vi "Read ODrive return data.vi"(8 "error in (no error)":errorcluster, 11 "Refnum in":refnum<k20>) -> (0 "error out":errorcluster, 3 "Refnum out":refnum<k20>)   [LabVIEW 2016]
uses:
  <vilib>/Utility/error.llb/Error Cluster From Error Code.vi
  <vilib>/RVI Host/nirviSupport.llb/nirviErrorClusterFromErrorCode.vi
  <vilib>/rvi/errors/niLvFpgaAdjustHostInterfaceError.vi
  Shared resoruces/ODrive State and Info.vi
  Shared resoruces/Navigation Variables.vi
  <vilib>/rvi/interface/nirviMethod/nirviMethod.xnode
  <vilib>/ErrorRing/Error Ring.xnode
  <vilib>/rvi/interface/nirviReadWriteControl/nirviReadWriteControl.xnode
  Shared resoruces/Shared resources RT.lvlib
  NiFpgaLv.dll
  <vilib>/rvi/interface/Simulation/niFpgaSimulationCallBeginRW.vi
  <vilib>/FPGAPlugInAG/Dynamic/niLvFpga_AcknowledgeIrq_Dynamic.vi
  <vilib>/rvi/interface/nirviMethod/StockFPGA_InlinedMethodWaitForSingleIRQ.vi
  <vilib>/FPGAPlugInAG/Dynamic/niLvFpga_WaitOnIrq_Dynamic.vi
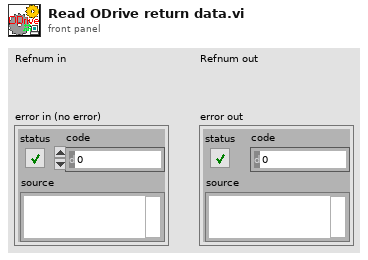
[diagram p1: front panel]
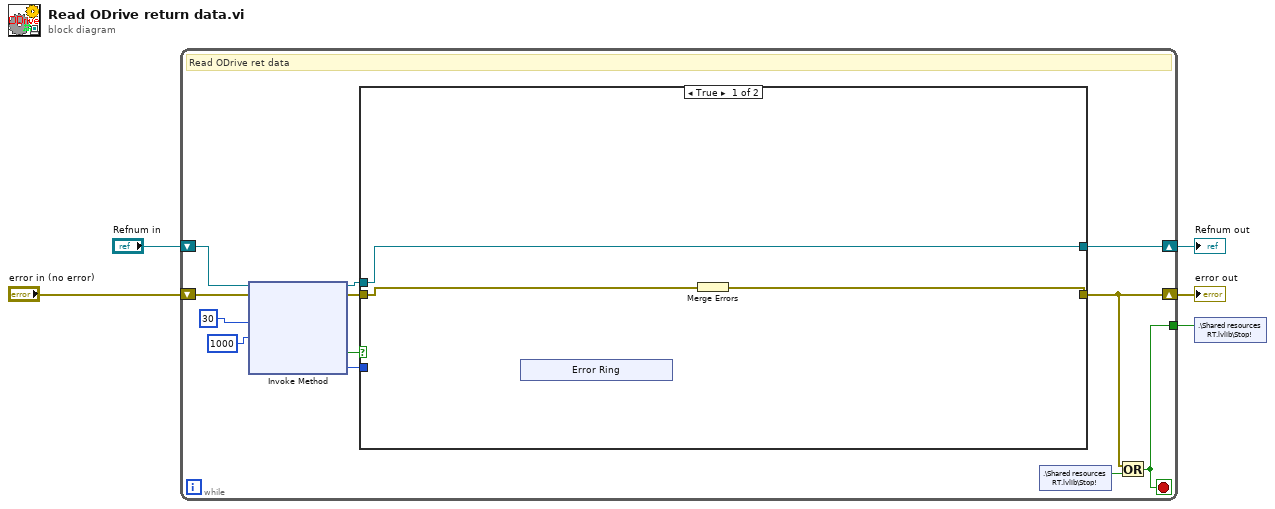
[diagram p0: block diagram]
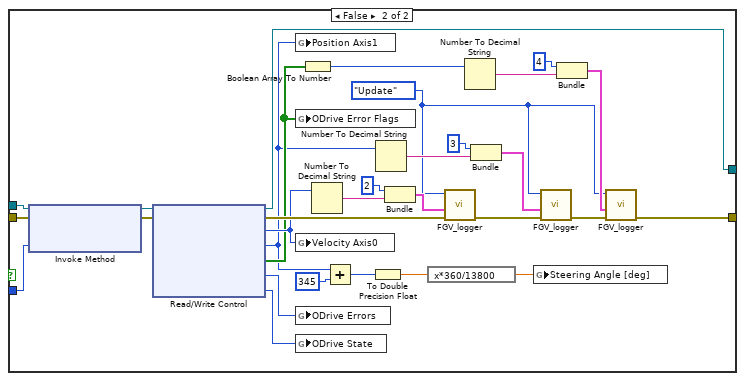
[diagram p2: hidden frame]
diagram:
  n1 = while {
    shift-right: [w17] -> w5
    shift-left: "Refnum in" -> [w16]
    shift-right: [w8] -> w2
    shift-left: "error in (no error)" -> [w15]
    tunnel: [w7] -> w1
    stop <- w7 stop-if-true
    # "Read ODrive ret data"
    n2 = xnode "Invoke Method"("FPGA VI Reference In"=w16, "error in"=w15, "IRQ Number(s)"=u8 30 ("Element"), "Timeout (ms)"=1000) -> ("FPGA VI Reference Out"=w12:refnum<k20>, "error out"=w13:errorcluster, "Timed Out"=w10:bool, "IRQ(s) Asserted"=w11:i32)
    n3 = case shown="True" w10 {
      tunnel: [w20 w55] -> w17
      tunnel: [w18 w40] -> w8
      tunnel: w13 -> [w19 w30]
      tunnel: w12 -> [w20 w29]
      tunnel: w11 -> [_ w26]
      frame True {
        n4 = xnode "Error Ring"() -> ()  [unwired: 1 out]
        n5 = Merge Errors(w19) -> (w18:errorcluster)
      }
      frame False {
        w42 = enum16{"Update", "Log", "Init"}."Update" ("Command")
        n6 = xnode "Invoke Method"("FPGA VI Reference In"=w29, "error in"=w30, "IRQ Number(s)"=w26) -> ("FPGA VI Reference Out"=w27:refnum<k20>, "error out"=w28:errorcluster)
        n7 = xnode "Read/Write Control"("FPGA VI Reference In"=w27, "error in"=w28) -> ("FPGA VI Reference Out"=w55:refnum<k20>, "error out"=w41:errorcluster, "Velocity Axis0"=w36:i16, "Position Axis1"=w34:i16, "ODrive Error Flags"=w35:bool[], "ODrive Errors"=w33:u32, "ODrive State"=w32:u8)
        n8 = global write "ODrive State and Info.vi" "Position Axis1"(w34) -> ()
        n9 = global write "ODrive State and Info.vi" "ODrive Error Flags"(w35) -> ()
        n10 = global write "ODrive State and Info.vi" "Velocity Axis0"(w36) -> ()
        n11 = global write "ODrive State and Info.vi" "ODrive Errors"(w33) -> ()
        n12 = global write "ODrive State and Info.vi" "ODrive State"(w32) -> ()
        n13 = Boolean Array To Number(Boolean array=w35) -> (number=w44:u8)
        n14 = Number To Decimal String(number=w36) -> (decimal integer string=w53:string)  [unwired: 1 in]
        n15 = Add(x=w34, y=i16 345 ("hi")) -> (x+y=w38:i16)
        n16 = To Double Precision Float(number=w38) -> (double precision float=w37:dbl)
        n17 = Number To Decimal String(number=w34) -> (decimal integer string=w50:string)  [unwired: 1 in]
        n18 = Bundle(2, w53) -> (w52:cluster{i32, string})  [unwired: 1 in]
        n19 = expression code="x*360/13800"(w37) -> (w31:dbl)
        n20 = call "FGV_logger.vi"("error in"=w41, 9:w52, "Command"=w42) -> ("error out"=w48:errorcluster)  [unwired: 8 in]
        n21 = Number To Decimal String(number=w44) -> (decimal integer string=w46:string)  [unwired: 1 in]
        n22 = Bundle(3, w50) -> (w49:cluster{i32, string})  [unwired: 1 in]
        n23 = global write "Navigation Variables.vi" "Steering Angle [deg]"(w31) -> ()
        n24 = call "FGV_logger.vi"("error in"=w48, 9:w49, "Command"=w42) -> ("error out"=w43:errorcluster)  [unwired: 8 in]
        n25 = Bundle(4, w46) -> (w45:cluster{i32, string})  [unwired: 1 in]
        n26 = call "FGV_logger.vi"("error in"=w43, 9:w45, "Command"=w42) -> ("error out"=w40:errorcluster)  [unwired: 8 in]
      }
    }
    n27 = shared-variable ".\\Shared resources RT.lvlib\\Stop!"() -> (w9:bool)  [unwired: 1 in, 1 out]
    n28 = Or(x=w8, y=w9) -> (x .or. y?=w7:bool)
  }
  "Refnum out" <- w5
  "error out" <- w2
  n29 = shared-variable ".\\Shared resources RT.lvlib\\Stop!"(w1) -> ()  [unwired: 1 in, 1 out]
